vi "Acquire CSV.vi"(8 "error in (no error)":errorcluster, 10 "DATA IN":refnum<queue>, 11 "Hardware Resources in":T1={"State"=enum."Idle S3DK", "Settings"="", "Online"=FALSE, "S3DK"={"Signals"={"Phasor"=[], "Analog"=[], "Digital"=[]}}, "CSV"={"CSV Path"=path "", "Index"=0, "Parcel Length"=0, "EOF?"=FALSE}}) -> (0 "error out":errorcluster, 3 "Hardware Resources out":T1={"State"=enum."Idle S3DK", "Settings"="", "Online"=FALSE, "S3DK"={"Signals"={"Phasor"=[], "Analog"=[], "Digital"=[]}}, "CSV"={"CSV Path"=path "", "Index"=0, "Parcel Length"=0, "EOF?"=FALSE}})   [LabVIEW 2017, in "Acquisition.lvlib"]
doc: "Perform the acquisition. Replace the contents of this diagram with calls to acquisition hardware."
uses:
  Acquisition.lvlib
  Acquisition Settings.ctl
  Acquisition State.ctl
  support/libs/PMU Buffer/Buffer DATA cluster.ctl
  <vilib>/Utility/file.llb/Read Delimited Spreadsheet (DBL).vi
  support/libs/PMU Buffer/PMU data buffer.lvlib
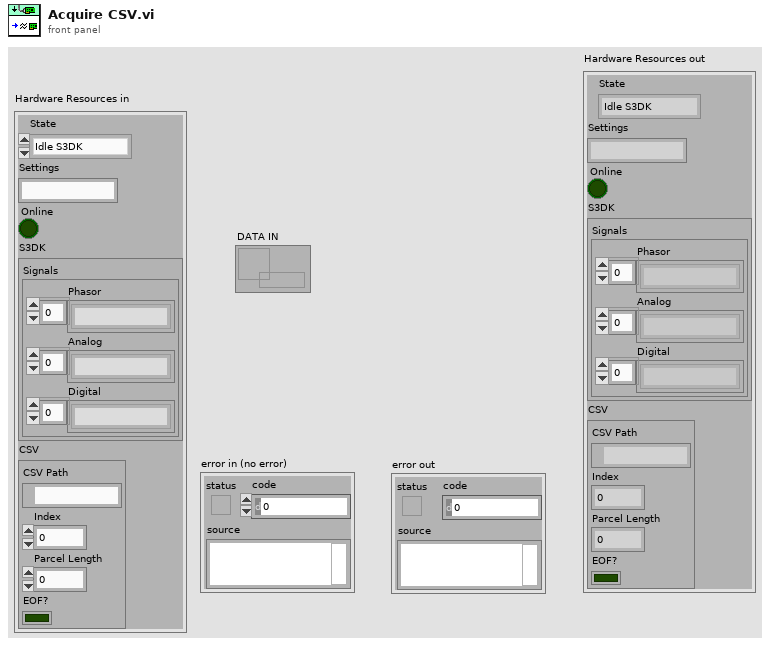
[diagram p1: front panel]
types:
  T1 = typedef "Acquisition.lvlib/Acquisition Settings.ctl" = cluster{"State":T2, "Settings":string, "Online":bool, "S3DK":cluster{"Signals":cluster{"Phasor":string[], "Analog":string[], "Digital":string[]}}, "CSV":cluster{"CSV Path":path, "Index":i32, "Parcel Length":i32, "EOF?":bool}}
  T2 = typedef "Acquisition.lvlib/Acquisition State.ctl" = enum16{"Idle", "Idle S3DK", "Acquiring S3DK", "Idle CSV", "Acquiring CSV"}
  T3 = typedef "PMU data buffer.lvlib/Buffer DATA cluster.ctl" = cluster{timestamp, csg[], sgl[]}
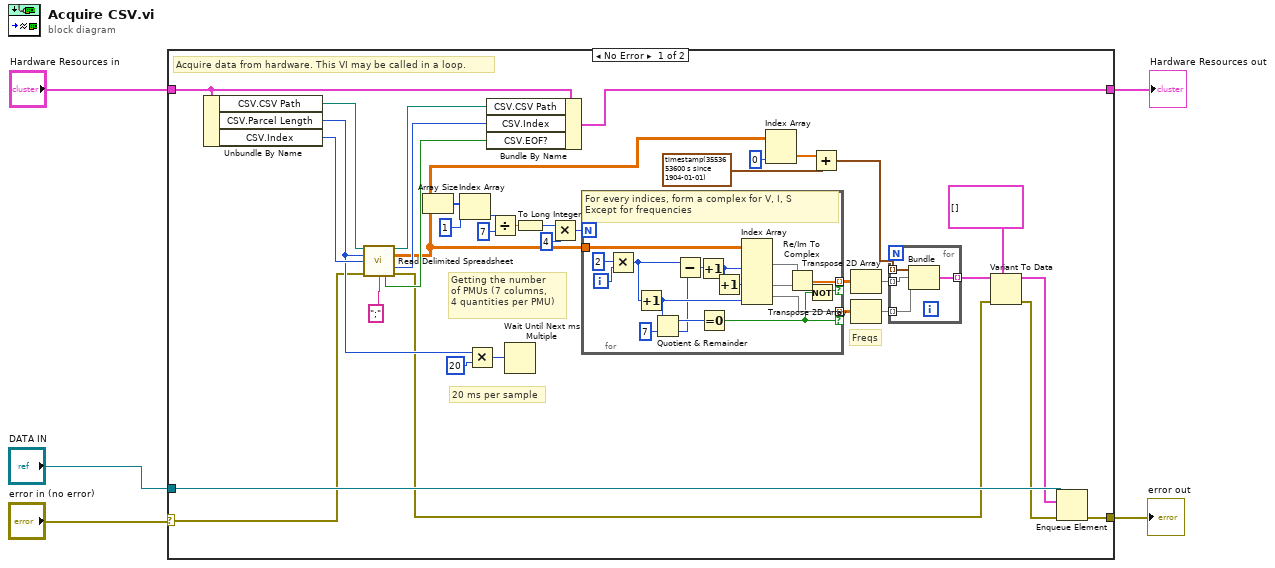
[diagram p0: block diagram]
diagram:
  n1 = case shown="No Error" "error in (no error)" {
    selector: "error in (no error)" -> [w6 w63]
    tunnel: [w40 w63] -> w4
    tunnel: "Hardware Resources in" -> [w36 w64]
    tunnel: [w33 w64] -> w2
    tunnel: "DATA IN" -> [w41 _]
    frame No Error {
      # "Freqs"
      # "Getting the number\nof PMUs (7 columns, \n4 quantities per PMU)"
      # "Acquire data from hardware. This VI may be called in a loop."
      # "20 ms per sample"
      n2 = Unbundle By Name(w36) -> ("CSV.CSV Path"=w35:path, "CSV.Parcel Length"=w27:i32, "CSV.Index"=w34:i32)
      n3 = call-poly <vilib>:"Read Delimited Spreadsheet.vi"("file path (dialog if empty)"=w35, "number of rows (all:-1)"=w27, "start of read offset (chars.:0)"=w34, "error in (no error)"=w6, "delimiter (\\t)"=";" ("delimiter (\\t)")) -> ("new file path (Not A Path if cancelled)"=w8:path, "all rows"=w18:dbl[][], "mark after read (chars.)"=w31:i32, "EOF?"=w32:bool, "error out"=w7:errorcluster)  [unwired: 5 in, 1 out]
      n4 = Array Size(array=w18) -> (size(s)=w21:i32[])
      n5 = Index Array(array=w21, index=1) -> (element=w23:i32)
      n6 = Multiply(x=w27, y=20) -> (x*y=w28:i32)
      n7 = Bundle By Name(cluster=w36, "CSV.CSV Path"=w8, "CSV.Index"=w31, "CSV.EOF?"=w32) -> (w33:T1)
      n8 = Divide(x=w23, y=7) -> (x/y=w25:dbl)
      n9 = Wait Until Next ms Multiple(millisecond multiple=w28) -> ()  [unwired: 1 out]
      n10 = To Long Integer(number=w25) -> (32bit integer=w9:i32)
      n11 = Multiply(x=w9, y=4) -> (x*y=w20:i32)
      n12 = for {
        N: w20 -> [_]
        tunnel: [w60] -> w13 mode=indexing if=w50
        tunnel: w18 -> [w57]
        tunnel: [w51] -> w12 mode=indexing if=w49
        i -> [w53]
        # "For every indices, form a complex for V, I, S\nExcept for frequencies"
        n13 = Multiply(x=2, y=w53) -> (x*y=w46:i32)
        n14 = Increment(x=w46) -> (x+1=w52:i32)
        n15 = Quotient & Remainder(x=w52, y=7) -> (x-y*floor(x/y)=w54:i32, floor(x/y)=w47:i32)
        n16 = Subtract(x=w46, y=w47) -> (x-y=w48:i32)
        n17 = Increment(x=w48) -> (x+1=w58:i32)
        n18 = Equal To 0?(x=w54) -> (x = 0?=w49:bool)
        n19 = Increment(x=w58) -> (x+1=w56:i32)
        n20 = Index Array(array=w57, index (col) #1=w58, index (col) #2=w56, index (col) #3=w52) -> (element #1=w61:dbl[], element #2=w62:dbl[], element #3=w51:dbl[])  [unwired: 3 in]
        n21 = Re/Im To Complex(1:w62, 2:w61) -> (0:w60:cdb[])
        n22 = Not(x=w49) -> (.not. x?=w50:bool)
      }
      n23 = Index Array(array=w18, index (col)=0 ("disabled index (col)")) -> (element=w17:dbl[])  [unwired: 1 in]
      n24 = Add(x=w17, y=timestamp(3553653600 s since 1904-01-01)) -> (x+y=w11:timestamp[])
      n25 = Transpose 2D Array(2D array=w13) -> (transposed array=w14:cdb[][])
      n26 = Transpose 2D Array(2D array=w12) -> (transposed array=w15:dbl[][])
      n27 = for {
        tunnel: w14 -> [w44] mode=indexing
        tunnel: w15 -> [w43] mode=indexing
        tunnel: w11 -> [w45] mode=indexing
        tunnel: [w42] -> w10 mode=indexing
        n28 = Bundle("Numeric"=w45, w44, w43) -> (w42:cluster{"Numeric":timestamp, cdb[], dbl[]})  [unwired: 1 in]
      }
      n29 = Variant To Data(error in=w7, type=T3[] [], Variant=w10) -> (data=w38:T3[], error out=w37:errorcluster)
      n30 = Enqueue Element(queue=w41, element=w38, error in (no error)=w37) -> (error out=w40:errorcluster)  [unwired: 1 in, 2 out]
    }
    frame Error {
    }
  }
  "Hardware Resources out" <- w2
  "error out" <- w4
